vi "poly_robust_unset_cursor_busy_state.vi"(8 "error in (no error)":errorcluster, 9 "disable click? (T)":bool=TRUE) -> (0 "error out":errorcluster, 1 "front pannel is closed?":bool)   [LabVIEW 2015]
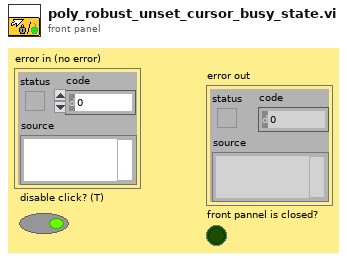
[diagram p1: front panel]
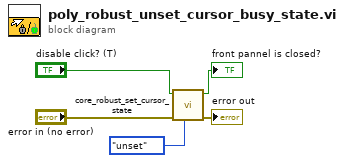
[diagram p0: block diagram]
diagram:
  n1 = call "core_robust_set_cursor_state.vi"("set/unset (set)"=enum16{"set", "unset"}."unset", "error in (no error)"="error in (no error)", "disable click? (T)"="disable click? (T)") -> ("error out"=→"error out":errorcluster, "front pannel is closed?"=→"front pannel is closed?":bool)  [unwired: 7 in]
